vi "bh3_stop_all_transmit_state.vi"(8 "error in (no error)":errorcluster, 11 "bt connection ID in":refnum<k31>) -> (0 "error out":errorcluster, 3 "bt connection ID out":refnum<k31>)   [LabVIEW 2013]
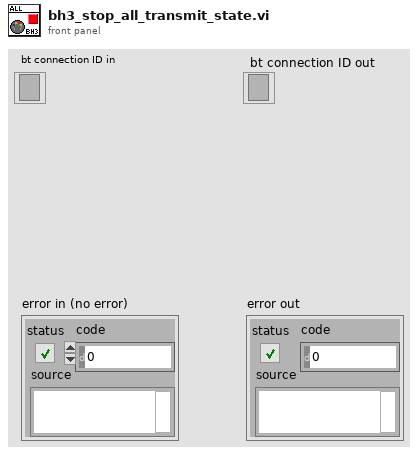
[diagram p1: front panel]
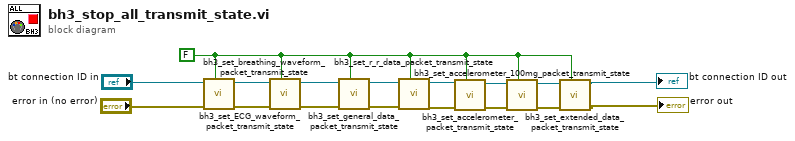
[diagram p0: block diagram]
diagram:
  w1 = FALSE ("enable?")
  n1 = call "bh3_set_breathing_waveform_packet_transmit_state.vi"("enable?"=w1, "error in (no error)"="error in (no error)", "bt connection ID in"="bt connection ID in") -> ("error out"=w15:errorcluster, "bt connection ID out"=w14:refnum<k31>)  [unwired: 7 in]
  n2 = call "bh3_set_ECG_waveform_packet_transmit_state.vi"("enable?"=w1, "error in (no error)"=w15, "bt connection ID in"=w14) -> ("error out"=w13:errorcluster, "bt connection ID out"=w12:refnum<k31>)  [unwired: 7 in]
  n3 = call "bh3_set_general_data_packet_transmit_state.vi"("enable?"=w1, "error in (no error)"=w13, "bt connection ID in"=w12) -> ("error out"=w11:errorcluster, "bt connection ID out"=w10:refnum<k31>)  [unwired: 7 in]
  n4 = call "bh3_set_r_r_data_packet_transmit_state.vi"("enable?"=w1, "error in (no error)"=w11, "bt connection ID in"=w10) -> ("error out"=w9:errorcluster, "bt connection ID out"=w8:refnum<k31>)  [unwired: 7 in]
  n5 = call "bh3_set_accelerometer_packet_transmit_state.vi"("enable?"=w1, "error in (no error)"=w9, "bt connection ID in"=w8) -> ("error out"=w7:errorcluster, "bt connection ID out"=w6:refnum<k31>)  [unwired: 7 in]
  n6 = call "bh3_set_accelerometer_100mg_packet_transmit_state.vi"("enable?"=w1, "error in (no error)"=w7, "bt connection ID in"=w6) -> ("error out"=w5:errorcluster, "bt connection ID out"=w4:refnum<k31>)  [unwired: 7 in]
  n7 = call "bh3_set_extended_data_packet_transmit_state.vi"("enable?"=w1, "error in (no error)"=w5, "bt connection ID in"=w4) -> ("error out"=→"error out":errorcluster, "bt connection ID out"=→"bt connection ID out":refnum<k31>)  [unwired: 7 in]
